vi "GetStepsPath.vi"(8 "error in (no error)":errorcluster) -> (0 "error out":errorcluster, 3 "Steps Folder Path":path)   [LabVIEW 2015, in "Configuration Tool.lvlib"]
uses:
  Configuration Tool.lvlib
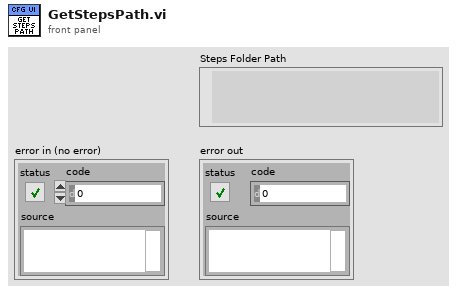
[diagram p1: front panel]
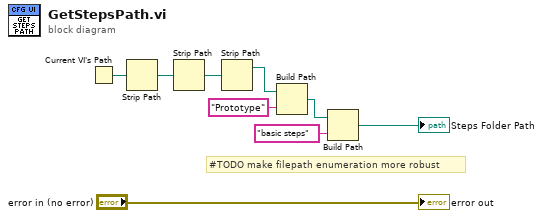
[diagram p0: block diagram]
diagram:
  # "#TODO make filepath enumeration more robust"
  n1 = Current VI's Path() -> (path=w8:path)
  n2 = Strip Path(path=w8) -> (stripped path=w2:path)  [unwired: 1 out]
  n3 = Strip Path(path=w2) -> (stripped path=w1:path)  [unwired: 1 out]
  n4 = Strip Path(path=w1) -> (stripped path=w7:path)  [unwired: 1 out]
  n5 = Build Path(base path=w7, name or relative path="Prototype") -> (appended path=w5:path)
  n6 = Build Path(base path=w5, name or relative path="basic steps") -> (appended path=→"Steps Folder Path":path)
  "error out" <- "error in (no error)"
